vi "GT Follow Data.vi"(5 "fifo":i16, 6 "type":i16, 7 "slaveSegment":dbl, 8 "error in (no error)":errorcluster caption="错误输入（无错误）", 9 "masterSegment":i32, 10 "profile":i16, 11 "cardNum":i16) -> (0 "error out":errorcluster caption="错误输出", 3 "function return":i16)   [LabVIEW 2020, in "gts.lvlib"]
doc: "GT_API GT_FollowData(short cardNum,short profile,long masterSegment,double slaveSegment,short type=FOLLOW_SEGMENT_NORMAL,short fifo=0);"
uses:
  gts.lvlib
  dll/32bit/multi_card/gts.dll
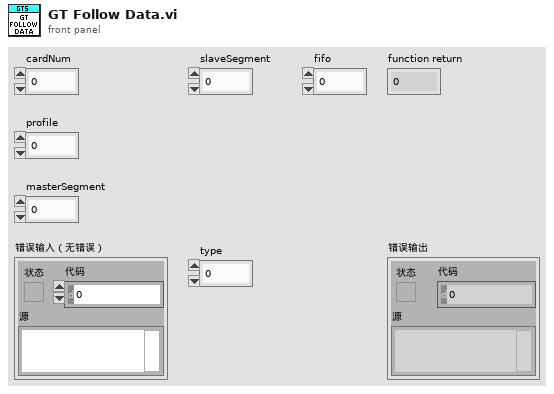
[diagram p1: front panel]
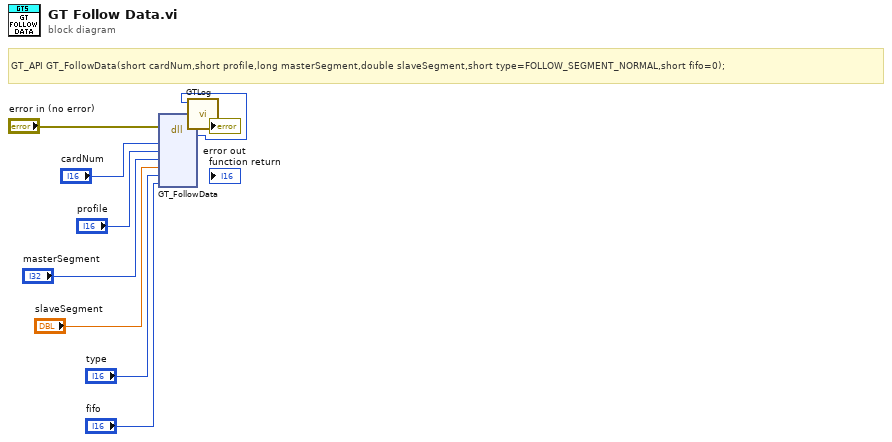
[diagram p0: block diagram]
diagram:
  # "GT_API GT_FollowData(short cardNum,short profile,long masterSegment,double slaveSegment,short type=FOLLOW_SEGMENT_NORMAL,short fifo=0);"
  n1 = dll-call lib="C:/1228/dll/32bit/multi_card/gts.dll" fn="GT_FollowData"(error in="error in (no error)", "cardNum"="cardNum", "profile"="profile", "masterSegment"="masterSegment", "slaveSegment"="slaveSegment", "type"="type", "fifo"="fifo") -> (error out=w3:errorcluster, w1:i16)  [unwired: 8 in, 1 out]
  n2 = call "GTLog.vi"("error in (no error)"=w3, "Numeric"=w1) -> ("error out"=→"error out":errorcluster)  [unwired: 9 in]
